vi "SubPanel_DataCollection_Rev11_v12.vi"(0 "DCPowerInformationClusterArray_Input":T7(array[cluster]), 1 "VISAPowerInfoInputArray":T6(array[cluster]), 2 "Run Data SubPanel Input":T5, 3 "RF Block Input Array":T1[](array[typedef]), 4 "Oscilloscope Info Array":T4(array[cluster]) {"vertical coupling" items=["AC", "DC", "Ground"]}, 6 "New Run?":bool, 7 "error in":errorcluster) -> (20 "DCPowerInformationClusterArray_Output":T7(array[cluster]), 21 "VISAPowerInfoInputOutput":T6(array[cluster]), 22 "Run Data SubPanel Output":T5, 23 "RF Subpanel Output":T1[](array[typedef]), 24 "Oscilloscope Info Array Output":T4(array[cluster]) {"vertical coupling" items=["AC", "DC", "Ground"]}, 25 "Reinitialize?":bool, 26 "Data Was Collected?":bool, 27 "error out":errorcluster)   [LabVIEW 2019]
uses:
  Controls/DataBlockControl.ctl
  Controls/QueueDataControl_V3.ctl
  <vilib>/Utility/file.llb/Write Delimited Spreadsheet (string).vi
  Controls/RFBlockControl.ctl
  <instrlib>/niScope/Controls/niScope vertical coupling.ctl
panel:
  out "RFSourceInfoArray":string[][](array[string])
  out "OscilloscopeInfoArray":string[][](array[string])
  out "Voltage Waveform Array":waveform(dbl)[](array[waveform])
  out "Current Waveform Array":waveform(dbl)[](array[waveform])
  out "Current Measurements Live":T2(graph)
  out "Voltage Measurements Live":T2(graph)
  out "DCPowerInfoArray":string[][](array[string])
  out "Current Measurements Total":cluster{dbl[], dbl[]}[](graph)
  out "Voltage Measurements Total":cluster{dbl[], dbl[]}[](graph)
  out "Exiting":bool
  out "Full Run Information":string
  out "Ready For Next Run?":bool
  in  "Next Run":bool
  out "Recording Data":bool
  in  "Record Data Toggle":bool
  out "error of collection":errorcluster
  in  "force exit SubVI":bool
  out "RF Block Parameters Output":T1
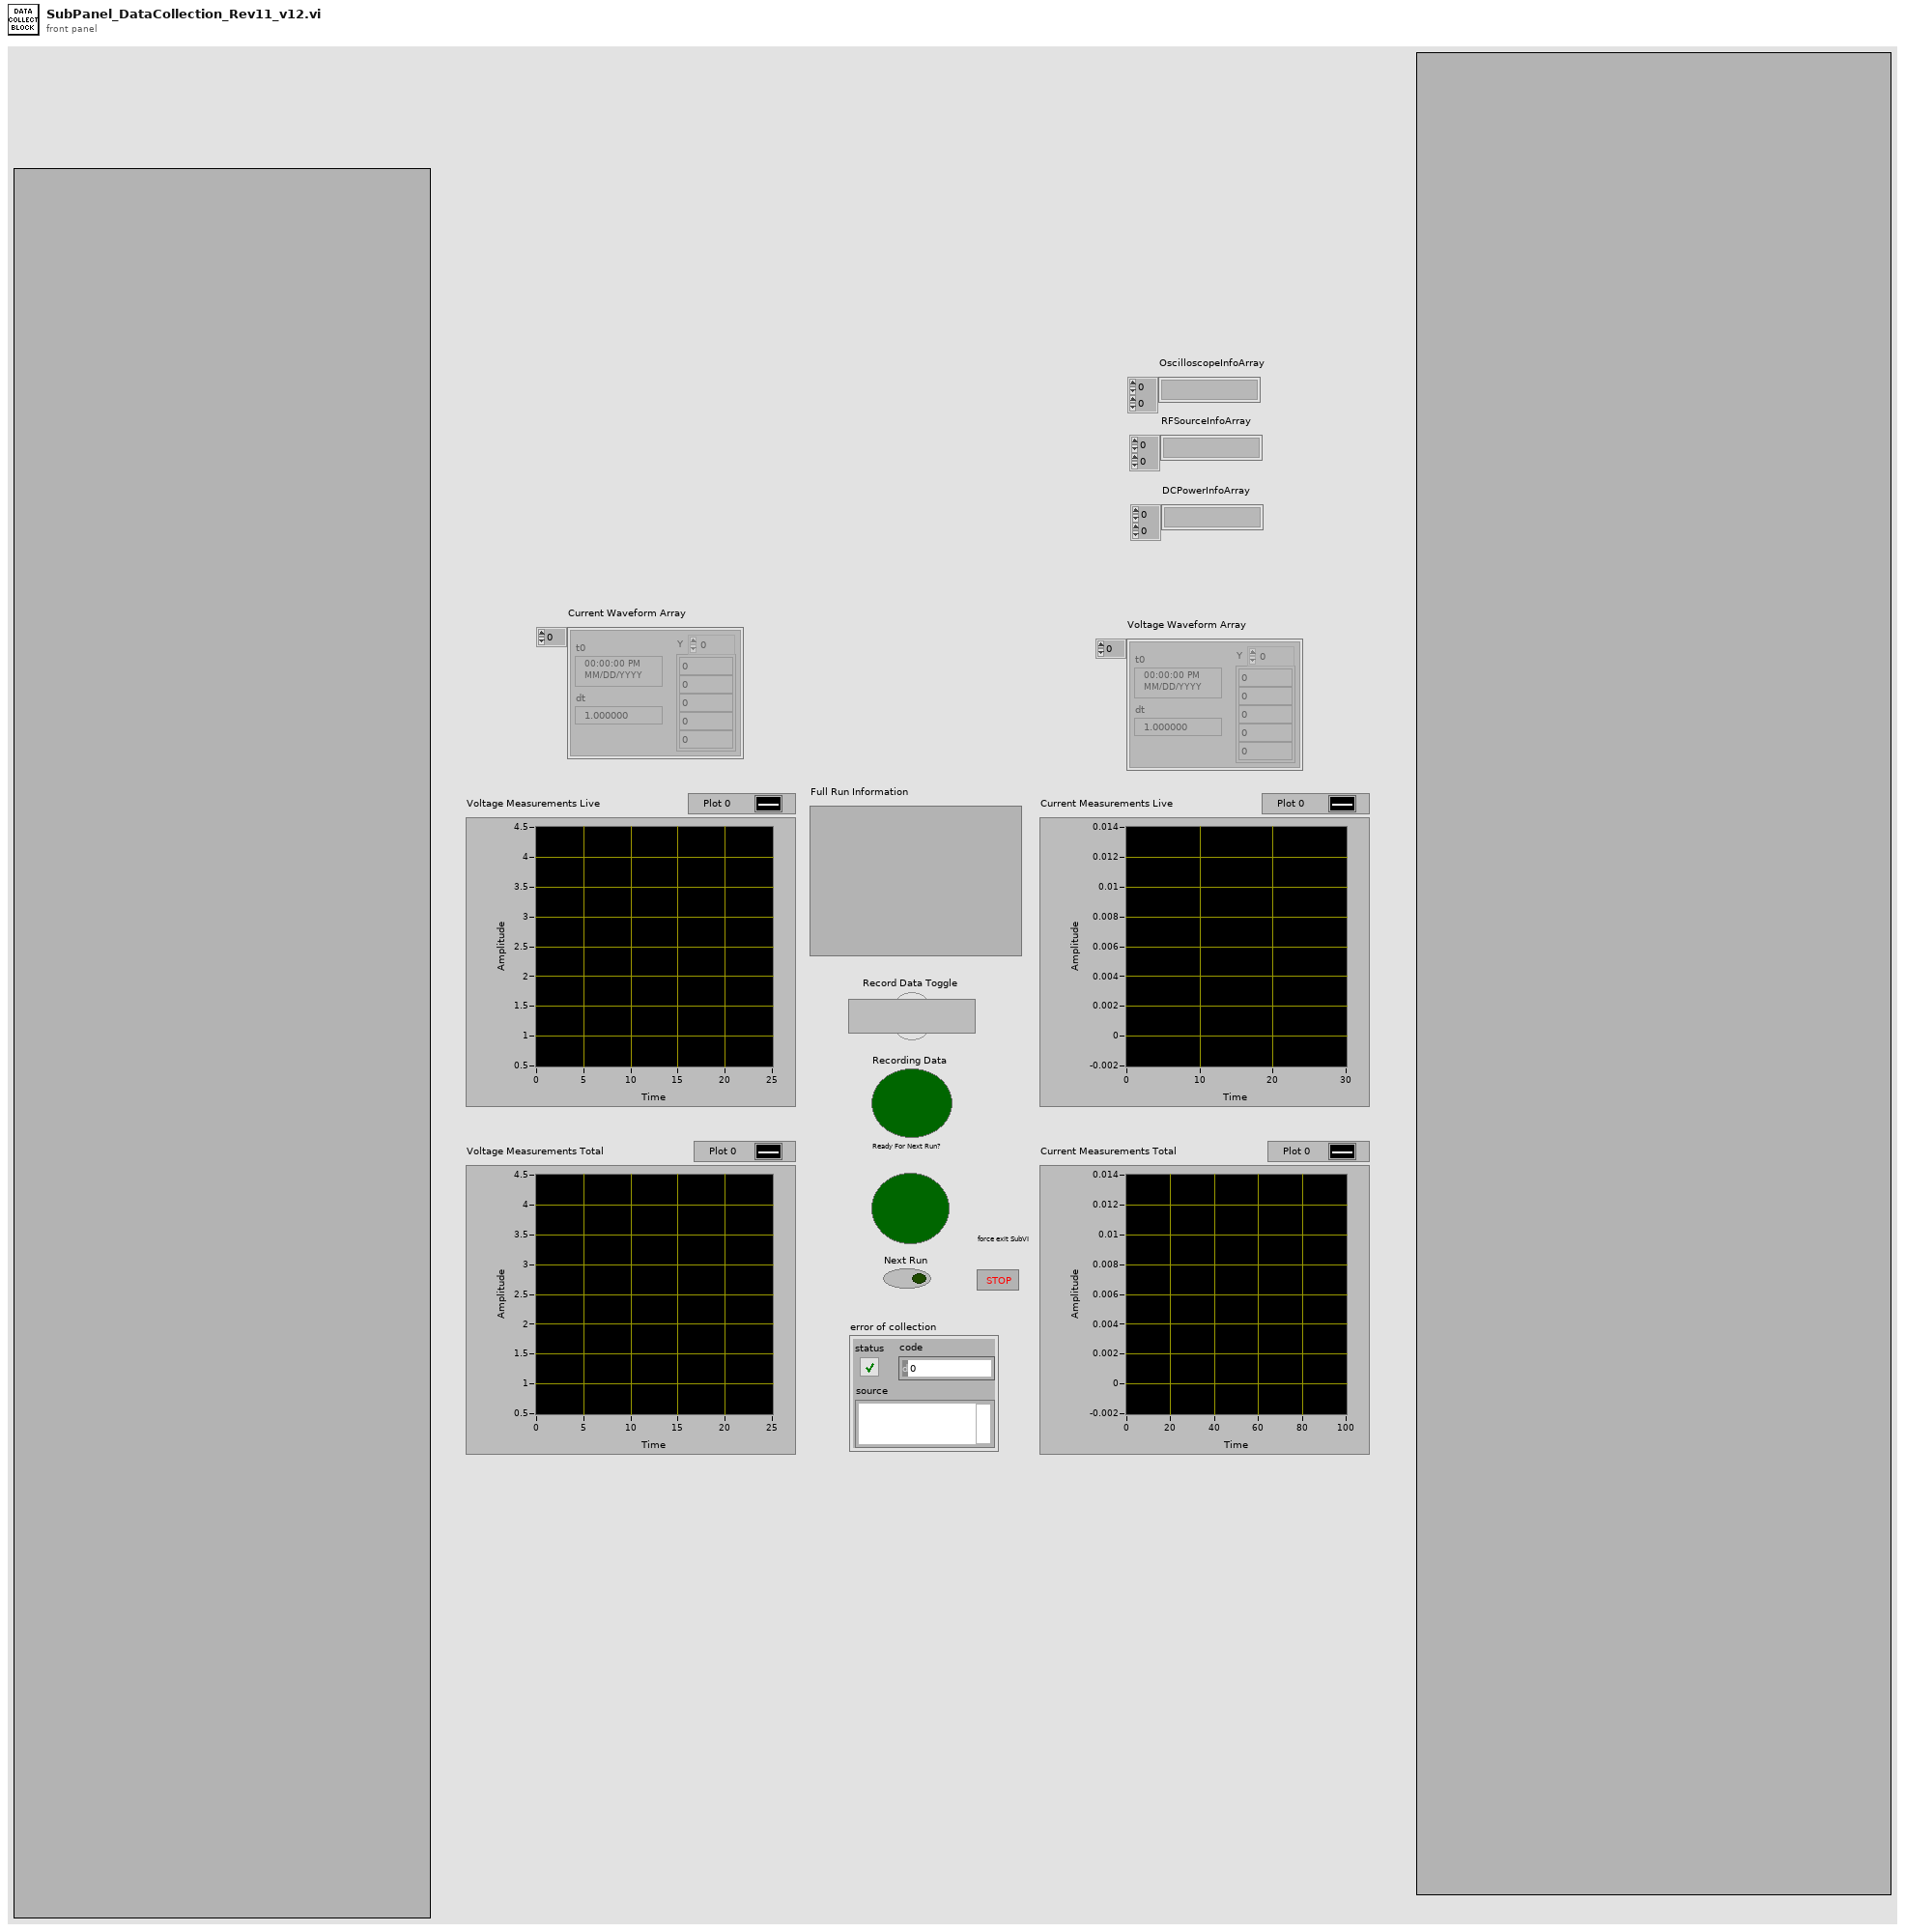
[diagram p1: front panel]
types:
  T1 = typedef "RFBlockControl.ctl" = cluster{"VISA resource name":refnum<visa-resource-name>, "RF Power State In":bool, "Frequency (GHz) Output":dbl, "Power (dBm) Output":dbl, "Instrument Name":string}
  T2 = cluster{"Array of fetched data":dbl[], "Array of fetched data":dbl[]}[]
  T3 = typedef "niScope vertical coupling.ctl" = i32
  T4 = cluster{"instrument handle out":refnum<k15>, "channel numbers array":string[], "channel names array":string[], "vertical range":dbl, "vertical coupling":T3, "Channel 0 50 ohms?":bool, "50 ohm vertical range (V)":dbl, "min record length":i32, "Actual Sample Rate":dbl}[]
  T5 = typedef "DataBlockControl.ctl" = cluster{"Run Folder Parent Directory":path, "DUT":string, "Ion (ex Kr)":string, "Board Number":string, "Effective LET":string, "Test Type":enum16{"Single Event Latchup", "Single Event Transient", "Single Event Upset"}}
  T6 = cluster{"VISA resource name":refnum<visa-resource-name>, "String List":string, string[], "Input Array (Voltage,Current_Limit)":dbl[], "Input Array (Voltage,Current_Limit)":dbl[], "Channel Names":string[], "read buffer":string}[]
  T7 = cluster{"instrument handle out":refnum<k15>, string, string[], dbl[], string[], "Current Limit Output Array":dbl[], dbl[]}[]
  T8 = enum16{"open", "replace", "create", "open or create", "replace or create", "replace or create with confirmation"}
  T9 = typedef "QueueDataControl_V3.ctl" = cluster{"Array of fetched data":dbl[][][], "Channel Names Array":string[], "Voltage Waveform Array":waveform(dbl)[], "Current Waveform Array":waveform(dbl)[], "Resetting Time":timestamp}
  T10 = cluster{"IVI Refnum out":refnum<k15>, string, "voltage level channel 23":dbl, "Channel Name 23":string, "Current Limit":dbl, "Measure Record dt":dbl, string}[]
  T11 = cluster{"created path":path, "DCPowerInformation_byChannel":cluster{"IVI Refnum out":refnum<k15>, string, "voltage level channel 23":dbl, "Channel Name 23":string, "Current Limit":dbl, "Measure Record dt":dbl, string}[], string[]}
  T12 = cluster{"Array of fetched data":dbl[][], string, i32[]}
  T13 = enum16{"Single Event Latchup", "Single Event Transient", "Single Event Upset"}
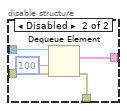
[diagram p3: hidden frame]
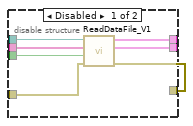
[diagram p5: hidden frame]
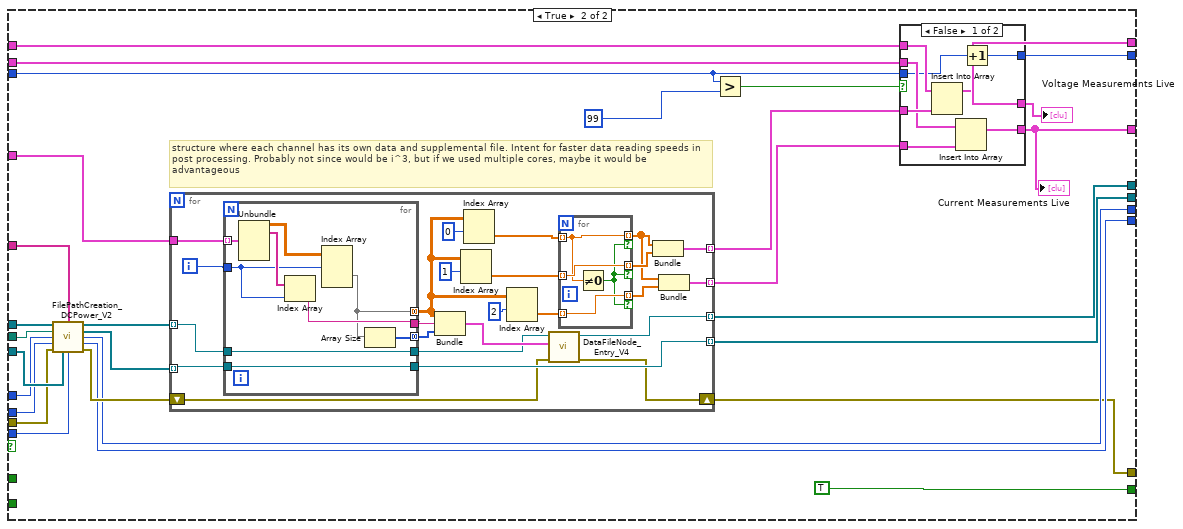
[diagram p6: hidden frame]
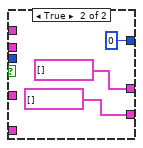
[diagram p7: hidden frame]
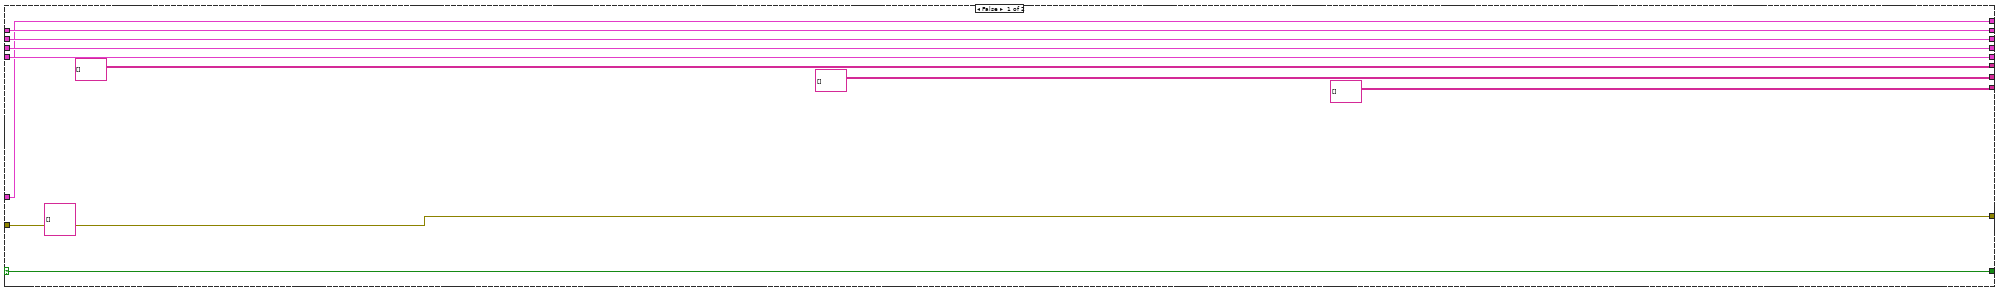
[diagram p8: hidden frame]
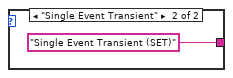
[diagram p9: hidden frame]
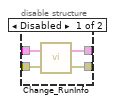
[diagram p13: hidden frame]
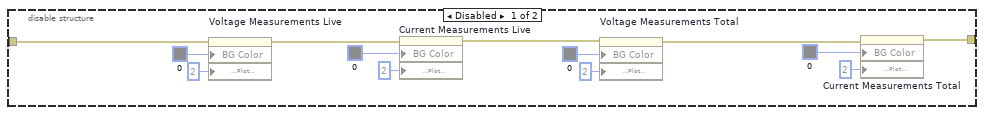
[diagram p14: hidden frame]
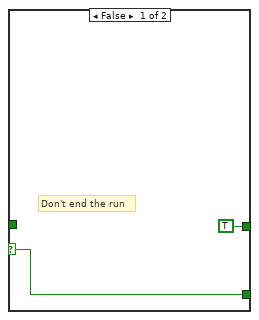
[diagram p16: hidden frame]
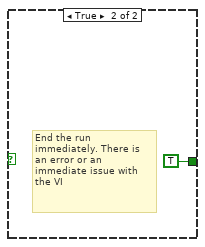
[diagram p17: hidden frame]
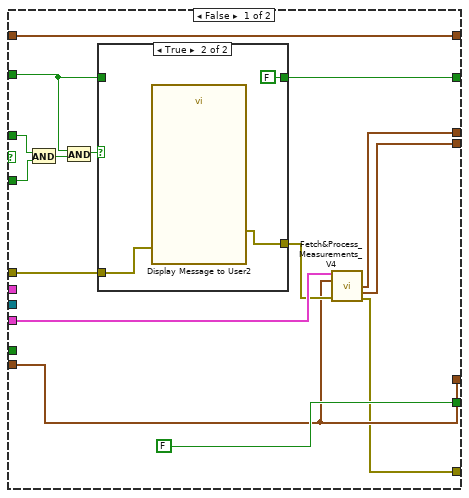
[diagram p19: hidden frame]
diagram:
  (unwired) string[] ["Instrument Name", "Channel Name", "Instrument Channel Number", "Voltage (V)", "Current Limit (A)", "Measure Record delta Time (s)"] ("new element/subarray")
  w76 = T9 {"Array of fetched data"=[], "Channel Names Array"=[], "Voltage Waveform Array"=[], "Current Waveform Array"=[], "Resetting Time"=timestamp(0 s since 1904-01-01)} ("DCPower Queue Data Double Array Format")
  (unwired) T9 {"Array of fetched data"=[], "Channel Names Array"=[], "Voltage Waveform Array"=[], "Current Waveform Array"=[], "Resetting Time"=timestamp(0 s since 1904-01-01)} ("DCPower Double Array Queue")
  (unwired) 10000 ("binary file indexor in")
  (unwired) T5 {"Run Folder Parent Directory"=path "", "DUT"="", "Ion (ex Kr)"="", "Board Number"="", "Effective LET"="", "Test Type"=enum."Single Event Latchup"} ("Run Data Configuration")
  # "Initiating the queue"
  # "echoing run information"
  # "Checking if this is a new run. If it is, a new folder is created along with references to a datafile node. If it is not new (i.e. you didn't start recording data because you needed to make a last minute change and pressed forced exit subvi), the previous folder that is theoretically empty (or just has the .txt files is used"
  # "If yes, you go into this subVI"
  # "This is the message at the beginning confirming if you want to make small changes to the program (i.e. LET)"
  # "Parameters from the configuration stage of this program"
  # "Reset the graph that is saving every 10 seconds of data. Every reset the low bound of the ten seconds is"
  # "Need to change to reflect number of channels that are being recorded. Collect this from a parameters file eventually that will be created"
  # "Indicator if the system is ready for another run. Also indicates if data was actually collected"
  # "Resets the system to start recording"
  # "A flag to ensure the warning message shows only once and doesn't lock the system"
  # "Initiating all of the DC Power instruments (doing this here so because we force abort channels in the DCPower setup because buffer overflow issues. Iterating over the instrument array and the active channel list"
  n1 = flat-sequence {
    tunnel: [w117] -> w92
    tunnel: "error in" -> [w107]
    tunnel: [w121] -> w97
    tunnel: "Run Data SubPanel Input" -> [w109]
    frame #0 {
      n2 = disable-structure shown="Enabled" {
        disable-tunnel: w107 -> [w134 w135]
        disable-tunnel: [w130 w135] -> w106
        frame Disabled {
          n3 = property on="Voltage Measurements Live" class="XYGraph (strict)"(error in=w134, "BG Color"=u32 0 ("Plot.Plot Color"), "Plot.Plot Interpolation"=u8 2) -> (error out=w133:errorcluster)  [unwired: 1 in, 1 out]
          n4 = property on="Current Measurements Live" class="XYGraph (strict)"(error in=w133, "BG Color"=u32 0 ("Plot.Plot Color"), "Plot.Plot Interpolation"=u8 2) -> (error out=w132:errorcluster)  [unwired: 1 in, 1 out]
          n5 = property on="Voltage Measurements Total" class="XYGraph (strict)"(error in=w132, "BG Color"=u32 0 ("Plot.Plot Color"), "Plot.Plot Interpolation"=u8 2) -> (error out=w131:errorcluster)  [unwired: 1 in, 1 out]
          n6 = property on="Current Measurements Total" class="XYGraph (strict)"(error in=w131, "BG Color"=u32 0 ("Plot.Plot Color"), "Plot.Plot Interpolation"=u8 2) -> (error out=w130:errorcluster)  [unwired: 1 in, 1 out]
        }
        frame Enabled {
        }
      }
      n7 = local write "Voltage Measurements Total"(cluster{dbl[], dbl[]}[] [] ("Voltage Measurements")) -> ()
      n8 = local write "Current Measurements Total"(cluster{dbl[], dbl[]}[] [] ("Current Measurements")) -> ()
      n9 = local write "Recording Data"(FALSE ("Recording Data")) -> ()
      n10 = local write "Exiting"(FALSE ("Forced Exit")) -> ()
      n11 = call "Convert_RunInfoCluster_2_RunInfoStringList.vi"("error in"=w106, "Run Number"="", "Run Data SubPanel Input"=w109) -> ("error output"=w110:errorcluster, "Run Data Output"=w111:string)
      n12 = call "Display Message to User"("error in (no error)"=w110, "Enable"=TRUE, "Message"=w111) -> ("error out"=w117:errorcluster)  [unwired: 7 in, 1 out]
      n13 = Two Button Dialog(message="Changing the LET?", 1:"No" ("F button name (\"Cancel\")"), 2:"Yes" ("T button name (\"OK\")")) -> (T button?=w121:bool)
    }
  }
  n14 = call "Convert_InstrumentReferenceArray_2_ChannelReferenceArray.vi"("error in (no error)"=w92, "DCPowerInformationClusterArray_Input"="DCPowerInformationClusterArray_Input") -> ("error out"=w91:errorcluster, "DCPowerInformation_byChannel"=w51:T10)
  n15 = case shown="True" w97 {
    tunnel: "Run Data SubPanel Input" -> [w137 w141]
    tunnel: [w137 w140] -> w29
    tunnel: [w136 w139] -> w93
    tunnel: w91 -> [w136 w138]
    frame False {
    }
    frame True {
      n16 = disable-structure shown="Enabled" {
        disable-tunnel: w141 -> [w145 w147]
        disable-tunnel: [w144 w146] -> w140
        disable-tunnel: [w143 w149] -> w139
        disable-tunnel: w138 -> [w142 w148]
        frame Disabled {
          n17 = call "Change_RunInfo.vi"("error in (no error)"=w142, "Run Data SubPanel in"=w145) -> ("error out"=w143:errorcluster, "Run Data SubPanel out"=w144:T5)
        }
        frame Enabled {
          n18 = call "Change_RunInfo_V2.vi"("error in (no error)"=w148, "Run Data SubPanel in"=w147) -> ("error out"=w149:errorcluster, "Run Data SubPanel out"=w146:T5)
        }
      }
    }
  }
  n19 = Unbundle(w29) -> ("Run Folder Parent Directory"=w94:path)  [unwired: 5 out]
  n20 = List Folder(path=w94, error in=w93) -> (folder names=w95:string[], error out=w79:errorcluster)  [unwired: 2 in, 2 out]
  n21 = Array Size(array=w95) -> (size(s)=w82:i32)
  n22 = case shown="True" "New Run?" {
    selector: "New Run?" -> [w151 w154]
    tunnel: [w152 w156] -> w83
    tunnel: w82 -> [w152 w155]
    tunnel: [w151 w154] -> w81
    tunnel: [w150 w153] -> w80
    tunnel: w79 -> [w150 w153]
    frame False {
    }
    frame True {
      n23 = Increment(x=w155) -> (x+1=w156:i32)
    }
  }
  n24 = Number To Decimal String(number=w83) -> (decimal integer string=w86:string)  [unwired: 1 in]
  n25 = Concatenate Strings("Run_", w86) -> (w28:string)
  n26 = Array Size(array=w51) -> (size(s)=w78:i32)
  n27 = call "InitialFileFolderCreation_V2.vi"("New Run?"=w81, "error in (no error)"=w80, "Run Number"=w28, "DCPowerArrayClusterSize"=w78, "base path"=w94) -> ("error out"=w27:errorcluster, "SupplementalDataFileReferenceObjectArray"=w89:refnum<file>[], "DataFileReferenceObjectArray"=w90:refnum<file>[], "created path"=w36:path)  [unwired: 3 in]
  n28 = call "Convert_RunInfoCluster_2_RunInfoStringList.vi"("error in"=w27, "Run Number"=w28, "Run Data SubPanel Input"=w29) -> ("error output"=w26:errorcluster, "Run Data Output"=→"Full Run Information":string)
  n29 = for {
    shift-right: [w157] -> w34
    shift-left: w26 -> [w159]
    tunnel: "DCPowerInformationClusterArray_Input" -> [w161] mode=indexing
    n30 = Unbundle(w161) -> ("instrument handle out"=w158:refnum<k15>, w160:string)  [unwired: 5 out]
    n31 = call <instrlib>:"niDCPower Initiate With Channels.vi"("error in (no error)"=w159, "channel name"=w160, "instrument handle"=w158) -> ("error out"=w157:errorcluster)  [unwired: 7 in, 1 out]
  }
  n32 = disable-structure shown="Enabled" {
    disable-tunnel: w34 -> [w165 w167]
    disable-tunnel: [w164 w167] -> w31
    disable-tunnel: [w163 _] -> w102
    disable-tunnel: w76 -> [w162 _]
    frame Enabled {
      n33 = Obtain Queue(name (unnamed)="DCPowerQueue", element data type=w162, error in (no error)=w165) -> (queue out=w163:refnum<queue>, error out=w164:errorcluster)  [unwired: 2 in, 1 out]
    }
    frame Disabled {
    }
  }
  n34 = disable-structure shown="Disabled" {
    frame Disabled {
      n35 = Reshape Array() -> ()  [unwired: 2 in, 1 out]
    }
    frame Enabled {
    }
  }
  n36 = for {
    tunnel: w51 -> [w169] mode=indexing
    tunnel: [w168] -> w52 mode=indexing
    # "Creating Array of Channel Names"
    n37 = Unbundle(w169) -> ("Channel Name 23"=w168:string)  [unwired: 6 out]
  }
  n38 = Bundle("created path"=w36, "DCPowerInformation_byChannel"=w51, w52) -> (w50:T11)  [unwired: 1 in]
  n39 = Array Size(array=w52) -> (size(s)=w71:i32)
  n40 = Get Date/Time In Seconds() -> (seconds since 1Jan1904=w32:timestamp)
  n41 = while {
    tunnel: w102 -> [w202]
    shift-right: [w189] -> w73
    shift-left: w31 -> [w201]
    tunnel: w36 -> [w198]
    shift-right: [w191] -> w75
    shift-left: w90 -> [w199]
    shift-right: [w190] -> w74
    shift-left: w89 -> [w197]
    shift-right: [w193] -> _
    shift-left: 0 ("binary file indexor in") -> [w196]
    shift-right: [w192] -> _
    shift-left: 0 ("binary file indexor in") -> [w195]
    tunnel: 1000 ("binary file indexor in") -> [w194]
    tunnel: w52 -> [w200]
    tunnel: w71 -> [_]
    shift-right: [w178] -> _
    shift-left: FALSE -> [w177]
    shift-right: [w174] -> _
    shift-left: T2 [] ("array") -> [w175]
    shift-right: [w172] -> _
    shift-left: T2 [] ("array") -> [w173]
    shift-right: [w170] -> _
    shift-left: 0 -> [w171]
    stop <- w186 stop-if-true
    # "If recording data is on, there should always be elements in the queue, so I shouldn't have to worry about a state where the \"recording data\" is active but there is no data in the queue, if so, then I'll just have to find an alternative to the OR statement"
    n42 = Get Queue Status(queue=w202, error in (no error)=w201) -> (queue out=w183:refnum<queue>, error out=w184:errorcluster, # elements in queue=w179:i32)  [unwired: 1 in, 5 out]
    n43 = local read "Recording Data"() -> (w176:bool)
    n44 = disable-structure shown="Enabled" {
      disable-tunnel: [w206 w208] -> w185
      disable-tunnel: w184 -> [w205 w210]
      disable-tunnel: w183 -> [w204 w211]
      disable-tunnel: [w203 w207] -> w182
      frame Enabled {
        n45 = Flush Queue(queue=w204, error in (no error)=w205) -> (remaining elements=w203:T9[], error out=w206:errorcluster)  [unwired: 1 out]
      }
      frame Disabled {
        n46 = Dequeue Element(queue=w211, timeout in ms (-1)=100, error in (no error)=w210) -> (element=w207:T9, error out=w208:errorcluster)  [unwired: 2 out]
      }
    }
    n47 = Not Equal To 0?(x=w179) -> (x != 0?=w181:bool)
    n48 = And(x=w181, y=w176) -> (x .and. y?=w180:bool)
    n49 = case shown="False" w180 {
      tunnel: w182 -> [_ w289]
      tunnel: w185 -> [w219 w283]
      tunnel: w200 -> [w220 w275]
      tunnel: w199 -> [w227 w288]
      tunnel: w198 -> [w221 w287]
      tunnel: w197 -> [w228 w286]
      tunnel: w196 -> [w226 w285]
      tunnel: w195 -> [w225 w274]
      tunnel: w194 -> [_ w273]
      tunnel: [w226 w282] -> w193
      tunnel: [w225 w281] -> w192
      tunnel: [w227 w278] -> w191
      tunnel: [w228 w277] -> w190
      tunnel: [w218 w276] -> w189
      tunnel: [w217 TRUE] -> w178
      tunnel: w177 -> [w216 _]
      tunnel: w176 -> [w224 _]
      tunnel: w175 -> [w215 w269]
      tunnel: [w215 w268] -> w174
      tunnel: w173 -> [w214 w267]
      tunnel: [w214 w266] -> w172
      tunnel: w171 -> [w213 w263]
      tunnel: [w212 w262] -> w170
      frame False {
        n50 = Not(x=w224) -> (.not. x?=w223:bool)
        n51 = And(x=w223, y=w216) -> (x .and. y?=w222:bool)
        n52 = case shown="True" w222 {
          tunnel: w221 -> [_ w240]
          tunnel: w220 -> [_ w239]
          tunnel: w219 -> [w231 w237]
          tunnel: [w231 w236] -> w218
          tunnel: [w230 FALSE] -> w217
          tunnel: w216 -> [w230 _]
          tunnel: w213 -> [w229 _]
          tunnel: [w229 0] -> w212
          frame False {
          }
          frame True {
            n53 = disable-structure shown="Enabled" {
              disable-tunnel: w240 -> [w247 w252]
              disable-tunnel: w239 -> [w246 w251]
              disable-tunnel: FALSE ("Create CSV files?") -> [w245 w253]
              disable-tunnel: w237 -> [w244 w254]
              disable-tunnel: [w243 _] -> w236
              disable-tunnel: [w242 w249] -> w234
              disable-tunnel: [w241 w248] -> w233
              frame Disabled {
                n54 = call "ReadDataFile_V1.vi"("error in (no error)"=w244, "Create CSV files?"=w245, "Channel Names Array"=w246, "DataFolder Path"=w247) -> ("error out"=w243:errorcluster, "Current Measurements"=w241:cluster{dbl[], dbl[]}[], "Voltage Measurements"=w242:cluster{dbl[], dbl[]}[])  [unwired: 5 in]
              }
              frame Enabled {
                n55 = Array Size(array=w251) -> (size(s)=w250:i32)
                n56 = for {
                  tunnel: w254 -> [w261]
                  tunnel: w253 -> [w260]
                  tunnel: w252 -> [w259]
                  tunnel: w251 -> [w258] mode=indexing
                  tunnel: w250 -> [w257]
                  tunnel: [w256] -> w249 mode=indexing
                  tunnel: [w255] -> w248 mode=indexing
                  n57 = call "ReadDataFile_V2.vi"("Channel Name Array Size"=w257, "error in (no error)"=w261, "Create CSV files?"=w260, "Channel Name Individual"=w258, "DataFolder Path"=w259) -> ("Current Measurements Individual"=w255:cluster{dbl[], dbl[]}, "Voltage Measurements Individual"=w256:cluster{dbl[], dbl[]})  [unwired: 4 in, 1 out]
                }
              }
            }
            "Voltage Measurements Total" <- w234
            "Current Measurements Total" <- w233
          }
        }
      }
      frame True {
        # "structure where each channel has its own data and supplemental file. Intent for faster data reading speeds in post processing. Probably not since would be i^3, but if we used multiple cores, maybe it would be advantageous"
        n58 = call "FilePathCreation_DCPower_V2.vi"("binary file input reference array 1"=w288, "Channel Name Input array"=w275, "data output directory folder"=w287, "binary file indexor in"=w285, "Reset counter in"=w274, "error in (no error)"=w283, "binary file input reference array 2"=w286, "reset threshold"=w273) -> ("binary file output reference array"=w280:refnum<file>[], "binary file output reference array 2"=w279:refnum<file>[], "binary file indexor out"=w282:i32, "reset counter out"=w281:i32, "error out"=w284:errorcluster)  [unwired: 3 in]
        n59 = for {
          shift-right: [w314] -> w276
          shift-left: w284 -> [w315]
          tunnel: w289 -> [w324]
          tunnel: w279 -> [w321] mode=indexing
          tunnel: w280 -> [w320] mode=indexing
          tunnel: [w319] -> w277 mode=indexing
          tunnel: [w313] -> w278 mode=indexing
          tunnel: [w308] -> w271 mode=indexing
          tunnel: [w307] -> w270 mode=indexing
          i -> [w318]
          n60 = for {
            tunnel: w324 -> [w337] mode=indexing
            tunnel: w318 -> [w334]
            tunnel: [w329] -> w309 mode=concatenating
            tunnel: [w333] -> w323
            tunnel: w321 -> [w332]
            tunnel: w320 -> [w330]
            tunnel: [w330] -> w316
            tunnel: [w332] -> w319
            tunnel: [w331] -> w322 mode=concatenating
            n61 = Unbundle(w337) -> ("Array of fetched data"=w336:dbl[][][], "Channel Names Array"=w335:string[])  [unwired: 3 out]
            n62 = Index Array(array=w335, index=w334) -> (element=w333:string)
            n63 = Index Array(array=w336, index (dim 0)=w334) -> (element=w329:dbl[][])  [unwired: 2 in]
            n64 = Array Size(array=w329) -> (size(s)=w331:i32[])
          }
          n65 = Bundle("Array of fetched data"=w309, w323, w322) -> (w317:T12)  [unwired: 1 in]
          n66 = Index Array(array=w309, index (row)=1) -> (element=w304:dbl[])  [unwired: 1 in]
          n67 = Index Array(array=w309, index (row)=0) -> (element=w306:dbl[])  [unwired: 1 in]
          n68 = Index Array(array=w309, index (row)=2) -> (element=w302:dbl[])  [unwired: 1 in]
          n69 = call "DataFileNode_Entry_V4.vi"("error in (no error)"=w315, "Queued Elements"=w317, "Byte Stream File in"=w316) -> ("error out"=w314:errorcluster, "Byte Stream File out"=w313:refnum<file>)  [unwired: 7 in]
          n70 = for {
            tunnel: [w326] -> w301 mode=indexing if=w325
            tunnel: w306 -> [w326] mode=indexing
            tunnel: [w328] -> w305 mode=indexing if=w325
            tunnel: w304 -> [w328] mode=indexing
            tunnel: [w327] -> w303 mode=indexing if=w325
            tunnel: w302 -> [w327] mode=indexing
            n71 = Not Equal To 0?(x=w326) -> (x != 0?=w325:bool)
          }
          n72 = Bundle(w301, w305) -> (w308:cluster{dbl[], dbl[]})  [unwired: 1 in]
          n73 = Bundle(w301, w303) -> (w307:cluster{dbl[], dbl[]})  [unwired: 1 in]
        }
        n74 = Greater?(x=w263, y=99) -> (0:w265:bool)
        n75 = case shown="False" w265 {
          tunnel: w271 -> [w297 _]
          tunnel: w270 -> [w296 _]
          tunnel: w269 -> [w295 _]
          tunnel: [w294 T2 [] ("array")] -> w268
          tunnel: w267 -> [w293 _]
          tunnel: [w292 T2 [] ("array")] -> w266
          tunnel: w263 -> [w291 _]
          tunnel: [w290 0] -> w262
          frame False {
            n76 = Insert Into Array(array=w295, new element=w297) -> (w294:T2)  [unwired: 1 in]
            n77 = Insert Into Array(array=w293, new element=w296) -> (w292:T2)  [unwired: 1 in]
            n78 = Increment(x=w291) -> (x+1=w290:i32)
          }
          frame True {
          }
        }
        "Voltage Measurements Live" <- w268
        "Current Measurements Live" <- w266
      }
    }
    n79 = local read "Exiting"() -> (w188:bool)
    n80 = Equal To 0?(x=w179) -> (x = 0?=w187:bool)
    n81 = And(x=w187, y=w188) -> (x .and. y?=w186:bool)
  }
  n82 = while {
    shift-right: [w368] -> w40
    shift-left: "DCPowerInformationClusterArray_Input" -> [w368]
    shift-right: [w372] -> w42
    shift-left: "VISAPowerInfoInputArray" -> [w372]
    shift-right: [w371] -> w44
    shift-left: w29 -> [w371]
    shift-right: [w370] -> w46
    shift-left: "RF Block Input Array" -> [w370]
    shift-right: [w369] -> w48
    shift-left: "Oscilloscope Info Array" -> [w369]
    shift-right: [w355] -> w77
    shift-left: w31 -> [w366]
    tunnel: w51 -> [w367]
    shift-right: [w365] -> _
    shift-left: FALSE -> [w362]
    tunnel: w102 -> [w364]
    shift-right: [w344] -> _
    shift-left: FALSE -> [w349]
    tunnel: [w353] -> w101
    shift-right: [w347] -> _
    shift-left: TRUE ("x .and. y?") -> [w348]
    shift-right: [w345] -> _
    shift-left: w32 -> [w346]
    tunnel: [w344] -> w39
    tunnel: w76 -> [w342]
    shift-right: [w339] -> w19
    shift-left: timestamp(0 s since 1904-01-01) ("seconds since 1Jan1904") -> [w338]
    stop <- w343 stop-if-true
    # "If I am going to reset the entire configuration or if we are going up in LET only. True, reset the system. False, don't reset the system"
    n83 = Not(x=w349) -> (.not. x?=w351:bool)
    n84 = And(x="Record Data Toggle", y=w351) -> (x .and. y?=w352:bool)
    "Recording Data" <- w352
    n85 = case shown="True" w352 {
      tunnel: w367 -> [w401 w416]
      tunnel: w366 -> [w399 w423]
      tunnel: [w389 w411] -> w341
      tunnel: [w390 w410] -> w340
      tunnel: w362 -> [_ w421]
      tunnel: [FALSE w422] -> w365
      tunnel: w364 -> [_ w420]
      tunnel: [w388 w419] -> w360
      tunnel: "Record Data Toggle" -> [w396 _]
      tunnel: w349 -> [w397 _]
      tunnel: w348 -> [w392 _]
      tunnel: [w393 TRUE] -> w347
      tunnel: w346 -> [w391 w424]
      tunnel: [w391 w414] -> w345
      tunnel: w342 -> [_ w418]
      tunnel: [w387 w408] -> w339
      tunnel: w338 -> [w387 w407]
      frame False {
        n86 = And(x=w396, y=w397) -> (x .and. y?=w395:bool)
        n87 = And(x=w392, y=w395) -> (x .and. y?=w394:bool)
        n88 = case shown="True" w394 {
          tunnel: [w403 w405] -> w398
          tunnel: w399 -> [w403 w406]
          tunnel: [w402 FALSE] -> w393
          tunnel: w392 -> [w402 _]
          frame False {
          }
          frame True {
            n89 = call "Display Message to User2"("error in (no error)"=w406) -> ("error out"=w405:errorcluster)  [unwired: 9 in, 1 out]
          }
        }
        n90 = call "Fetch&Process_Measurements_V4.vi"("DCPowerInformation_byChannel"=w401, "Initial Time"=w391, "error in (no error)"=w398) -> ("Current Waveform Array"=w389:waveform(dbl)[], "Voltage Waveform Array"=w390:waveform(dbl)[], "error out"=w388:errorcluster)  [unwired: 6 in, 4 out]
      }
      frame True {
        n91 = case shown="True" w421 {
          tunnel: [w426 w432] -> w414
          tunnel: w424 -> [_ w432]
          tunnel: w423 -> [w427 w431]
          tunnel: [w427 w431] -> w415
          tunnel: [TRUE w430] -> w422
          tunnel: w421 -> [_ w430]
          tunnel: [w426 w429] -> w408
          tunnel: w407 -> [_ w429]
          frame False {
            n92 = Get Date/Time In Seconds() -> (seconds since 1Jan1904=w426:timestamp)
          }
          frame True {
          }
        }
        n93 = call "Fetch&Process_Measurements_V4.vi"("DCPowerInformation_byChannel"=w416, "Initial Time"=w414, "error in (no error)"=w415) -> ("Data As dbl Array"=w413:dbl[][][], "Channel Number Array"=w412:string[], "Current Waveform Array"=w411:waveform(dbl)[], "Voltage Waveform Array"=w410:waveform(dbl)[], "error out"=w409:errorcluster)  [unwired: 6 in, 2 out]
        n94 = Bundle(cluster=w418, "Array of fetched data"=w413, "Channel Names Array"=w412) -> (w417:T9)  [unwired: 3 in]
        n95 = Enqueue Element(queue=w420, element=w417, error in (no error)=w409) -> (error out=w419:errorcluster)  [unwired: 1 in, 2 out]
      }
    }
    "Current Waveform Array" <- w341
    "Voltage Waveform Array" <- w340
    n96 = Not(x=w352) -> (.not. x?=w363:bool)
    n97 = And(x=w363, y=w362) -> (x .and. y?=w361:bool)
    n98 = case shown="True" w361 {
      tunnel: w360 -> [w383 w385]
      tunnel: [w384 TRUE] -> w344
      tunnel: w349 -> [w384 _]
      tunnel: [w383 w385] -> w355
      frame False {
      }
      frame True {
      }
    }
    "error of collection" <- w355
    "Ready For Next Run?" <- w344
    n99 = Or(x=w355, y="force exit SubVI") -> (x .or. y?=w357:bool)
    n100 = And(x="Next Run", y=w344) -> (x .and. y?=w359:bool)
    n101 = Or(x=w357, y=w359) -> (x .or. y?=w358:bool)
    n102 = case shown="True" w358 {
      selector: w358 -> [w374 _]
      tunnel: w357 -> [_ w377]
      tunnel: [w374 TRUE] -> w343
      tunnel: [TRUE ("T button?") w375] -> w353
      frame False {
        # "Don't end the run"
      }
      frame True {
        n103 = case shown="False" w377 {
          tunnel: [w378 TRUE] -> w375
          frame False {
            # "Option to continue the run as is or reset for a new configuration"
            n104 = Two Button Dialog(message="Would you like to change parameters before the next run? ( you will have an option to change LET and board number regardless) ", 1:"No, I may only want to change LET or board number" ("F button name (\"Cancel\")"), 2:"Yes, I want to make changes " ("T button name (\"OK\")")) -> (T button?=w378:bool)
          }
          frame True {
            # "End the run immediately. There is an error or an immediate issue with the VI"
          }
        }
      }
    }
    "Exiting" <- w343
  }
  "Reinitialize?" <- w101
  n105 = for {
    tunnel: w75 -> [w437] mode=indexing
    tunnel: w74 -> [w435] mode=indexing
    shift-right: [w433] -> w72
    shift-left: w73 -> [w436]
    n106 = Close File(refnum=w437, error in=w436) -> (error out=w434:errorcluster)  [unwired: 1 out]
    n107 = Close File(refnum=w435, error in=w434) -> (error out=w433:errorcluster)  [unwired: 1 out]
  }
  n108 = Merge Errors(w77, w72) -> (w54:errorcluster)
  n109 = Unbundle(w50) -> ("created path"=w35:path)  [unwired: 2 out]
  n110 = case shown="True" w39 {
    selector: w39 -> [w442 w547]
    tunnel: w54 -> [w441 w553]
    tunnel: [w441 w452] -> w53
    tunnel: [w447 w484] -> w49
    tunnel: w48 -> [w447 w552]
    tunnel: [w446 w486] -> w47
    tunnel: w46 -> [w446 w551]
    tunnel: [w445 w472] -> w45
    tunnel: w44 -> [w445 w550]
    tunnel: [w444 w489] -> w43
    tunnel: w42 -> [w444 w549]
    tunnel: [w443 w491] -> w41
    tunnel: w40 -> [w443 w548]
    tunnel: [w442 w547] -> w38
    tunnel: [string[][] [] ("DCPowerInfoArray") w482] -> w37
    tunnel: w35 -> [_ w450]
    tunnel: [string[][] [] ("DCPowerInfoArray") w480] -> w3
    tunnel: [string[][] [] ("DCPowerInfoArray") w474] -> w2
    frame False {
      (unwired) string[][][] []
    }
    frame True {
      # "This will be indexed eventually"
      n111 = for {
        shift-right: [w633] -> w543
        shift-left: w553 -> [w645]
        tunnel: w548 -> [w636] mode=indexing
        shift-right: [w644] -> w522
        shift-left: w552 -> [w644]
        shift-right: [w643] -> w521
        shift-left: w551 -> [w643]
        shift-right: [w642] -> w520
        shift-left: w550 -> [w642]
        shift-right: [w641] -> w519
        shift-left: w549 -> [w641]
        shift-right: [w640] -> w518
        shift-left: w548 -> [w640]
        shift-right: [w638] -> w523
        shift-left: string[][] [] ("DCPowerInfoArray") -> [w639]
        # "This puts all the instruments together in one output"
        n112 = Unbundle(w636) -> ("instrument handle out"=w647:refnum<k15>, w646:string)  [unwired: 5 out]
        n113 = call <instrlib>:"niDCPower Abort With Channels.vi"("error in (no error)"=w645, "channel name"=w646, "instrument handle"=w647) -> ("error out"=w634:errorcluster)  [unwired: 7 in, 1 out]
        n114 = call "DCPower_ParameterCreation.vi"("error in"=w634, "Precision"="8", "DCPowerInformationByInstrument"=w636) -> ("error out"=w633:errorcluster, "DCPowerInfoArray"=w632:string[][])
        n115 = Insert Into Array(array=w639, index (col)=0 ("disabled index (col)"), new element=w632) -> (w638:string[][])  [unwired: 1 in]
      }
      n116 = Concatenate Strings("Channel Name " ("string")) -> (w535:string)
      n117 = Concatenate Strings("Voltage (V) " ("string")) -> (w537:string)
      n118 = Concatenate Strings("Measure Record delta Time (s) " ("string")) -> (w539:string)
      n119 = Concatenate Strings("Instrument Name " ("string")) -> (w534:string)
      n120 = Concatenate Strings("Instrument Channel Number " ("string")) -> (w536:string)
      n121 = Concatenate Strings("Current Limit (A) " ("string")) -> (w538:string)
      n122 = Build Array(w534, w535, w536, w537, w538, w539) -> (w527:string[])
      n123 = Build Path(base path=w450, name or relative path="DCPOW_Params.csv") -> (appended path=w542:path)
      n124 = Insert Into Array(array=w523, index (col)=0 ("disabled index (col)"), new element=w527) -> (w526:string[][])  [unwired: 1 in]
      n125 = call-poly <vilib>:"Write Delimited Spreadsheet.vi"("file path (dialog if empty)"=w542, "format (%s)"="%s" ("format (%.3f)"), "2D data"=w526, "error in (no error)"=w543, "transpose? (no:F)"=TRUE, "delimiter (\\t)"="," ("delimiter (\\t)")) -> ("error out"=w524:errorcluster)  [unwired: 8 in, 1 out]
      n126 = for {
        shift-right: [w626] -> w504
        shift-left: w524 -> [w626]
        shift-right: [w621] -> w492
        shift-left: w518 -> [w621]
        shift-right: [w622] -> w490
        shift-left: w519 -> [w622]
        shift-right: [w623] -> w488
        shift-left: w520 -> [w623]
        shift-right: [w624] -> w487
        shift-left: w521 -> [w624]
        shift-right: [w625] -> w483
        shift-left: w523 -> [w625]
        tunnel: w522 -> [w620] mode=indexing
        tunnel: [w620] -> w485 mode=indexing
        shift-right: [w589] -> w481
        shift-left: string[][] [] ("DCPowerInfoArray") -> [w595]
        n127 = Unbundle(w620) -> ("instrument handle out"=w619:refnum<k15>, "channel numbers array"=w592:string[], "channel names array"=w593:string[], "vertical range"=w614:dbl, "vertical coupling"=w608:T3, "Channel 0 50 ohms?"=w613:bool, "50 ohm vertical range (V)"=w612:dbl, "min record length"=w607:i32, "Actual Sample Rate"=w606:dbl)
        n128 = Array Size(array=w592) -> (size(s)=w615:i32)
        n129 = Initialize Array(w614, w615) -> (w611:dbl[])
        n130 = Decimal String To Number(string="8") -> (number=w590:i32)  [unwired: 2 in, 1 out]
        n131 = case shown="True" w613 {
          tunnel: w612 -> [_ w629]
          tunnel: w611 -> [w627 w631]
          tunnel: [w627 w628] -> w610
          frame False {
          }
          frame True {
            n132 = Replace Array Subset(array=w631, new element=w629, index=0) -> (w628:dbl[])
          }
        }
        n133 = Number To Fractional String(number=w606, precision (6)=w590) -> (F-format string=w600:string)  [unwired: 2 in]
        n134 = Number To Decimal String(number=w607) -> (decimal integer string=w601:string)  [unwired: 1 in]
        n135 = Concatenate Strings(w619) -> (w617:string)
        n136 = Number To Fractional String(number=w610, precision (6)=w590) -> (F-format string=w609:string[])  [unwired: 2 in]
        n137 = Number To Decimal String(number=w608) -> (decimal integer string=w602:string)  [unwired: 1 in]
        n138 = Array Size(array=w592) -> (size(s)=w618:i32)
        n139 = Initialize Array(w617, w618) -> (w616:string[])
        n140 = Array Size(array=w592) -> (size(s)=w605:i32)
        n141 = Array Size(array=w592) -> (size(s)=w603:i32)
        n142 = Array Size(array=w592) -> (size(s)=w604:i32)
        n143 = Initialize Array(w602, w605) -> (w599:string[])
        n144 = Initialize Array(w600, w603) -> (w597:string[])
        n145 = Initialize Array(w601, w604) -> (w598:string[])
        n146 = Build Array(w616, w593, w592, w609, w599, w598, w597) -> (w594:string[][])
        n147 = Insert Into Array(array=w595, index (col)=0 ("disabled index (col)"), new element=w594) -> (w589:string[][])  [unwired: 1 in]
      }
      n148 = Build Array("Instrument Name " ("string"), "Channel Name" ("element"), "Instrument Channel Number" ("element"), "Vertical Range (V)" ("element"), "Vertical Coupling" ("element"), "Min Record Length" ("element"), "Actual Sample Rate" ("element")) -> (w508:string[])
      n149 = Insert Into Array(array=w481, index (col)=0 ("disabled index (col)"), new element=w508) -> (w501:string[][])  [unwired: 1 in]
      n150 = Build Path(base path=w450, name or relative path="Oscilloscope_Params.csv") -> (appended path=w506:path)
      n151 = call-poly <vilib>:"Write Delimited Spreadsheet.vi"("file path (dialog if empty)"=w506, "format (%s)"="%s" ("format (%.3f)"), "2D data"=w501, "error in (no error)"=w504, "transpose? (no:F)"=TRUE, "delimiter (\\t)"="," ("delimiter (\\t)")) -> ("error out"=w499:errorcluster)  [unwired: 8 in, 1 out]
      n152 = for {
        shift-right: [w571] -> w497
        shift-left: string[][] [] ("DCPowerInfoArray") -> [w572]
        tunnel: w487 -> [w587] mode=indexing
        shift-right: [w556] -> w473
        shift-left: w499 -> [w563]
        shift-right: [w564] -> w480
        shift-left: w481 -> [w564]
        shift-right: [w565] -> w482
        shift-left: w483 -> [w565]
        shift-right: [w566] -> w484
        shift-left: w485 -> [w566]
        shift-right: [w567] -> w486
        shift-left: w487 -> [w567]
        shift-right: [w568] -> w472
        shift-left: w488 -> [w568]
        shift-right: [w569] -> w489
        shift-left: w490 -> [w569]
        shift-right: [w570] -> w491
        shift-left: w492 -> [w570]
        n153 = Unbundle(w587) -> ("VISA resource name"=w586:refnum<visa-resource-name>, "Frequency (GHz) Output"=w580:dbl, "Power (dBm) Output"=w577:dbl)  [unwired: 2 out]
        n154 = Decimal String To Number(string="8") -> (number=w575:i32)  [unwired: 2 in, 1 out]
        n155 = VISA Write(VISA resource name=w586, write buffer="*IDN?", error in (no error)=w563) -> (VISA resource name out=w582:refnum<visa-resource-name>, return count=w584:u32, error out=w588:errorcluster)
        n156 = Number To Fractional String(number=w577, precision (6)=w575) -> (F-format string=w578:string)  [unwired: 2 in]
        n157 = Add(x=w584, y=u32 10) -> (x+y=w581:u32)
        n158 = Number To Fractional String(number=w580, precision (6)=w575) -> (F-format string=w579:string)  [unwired: 2 in]
        n159 = VISA Read(VISA resource name=w582, byte count=w581, error in (no error)=w588) -> (read buffer=w562:string, error out=w557:errorcluster)  [unwired: 2 out]
        n160 = Search and Replace String(replace all?=TRUE ("replace all? (F)"), input string=w562, search string=",", replace string="_" ("replace string (\"\")"), error in=w557) -> (result string=w559:string, error out=w556:errorcluster)  [unwired: 3 in, 2 out]
        n161 = Build Array(w559, w579, w578) -> (w574:string[])
        n162 = Insert Into Array(array=w572, index (col)=0 ("index (row)"), new element=w574) -> (w571:string[][])  [unwired: 1 in]
      }
      n163 = Build Array("Instrument Name", "Frequency (GHz)" ("element"), "Power (dBm)" ("element")) -> (w493:string[])
      n164 = Build Path(base path=w450, name or relative path="RFSource_Params.csv") -> (appended path=w478:path)
      n165 = Insert Into Array(array=w497, index (col)=0 ("disabled index (col)"), new element=w493) -> (w474:string[][])  [unwired: 1 in]
      n166 = call-poly <vilib>:"Write Delimited Spreadsheet.vi"("file path (dialog if empty)"=w478, "format (%s)"="%s" ("format (%.3f)"), "2D data"=w474, "error in (no error)"=w473, "transpose? (no:F)"=TRUE, "delimiter (\\t)"="," ("delimiter (\\t)")) -> ("error out"=w453:errorcluster)  [unwired: 8 in, 1 out]
      n167 = Strip Path(path=w450) -> (name=w471:string)  [unwired: 1 out]
      n168 = Unbundle(w472) -> ("DUT"=w470:string, "Ion (ex Kr)"=w469:string, "Board Number"=w468:string, "Effective LET"=w467:string, "Test Type"=w466:T13)  [unwired: 1 out]
      n169 = case shown="\"Single Event Latchup\", Default" w466 {
        tunnel: ["Single Event Latchup (SEL)" "Single Event Transient (SET)"] -> w465
        frame "Single Event Latchup", Default {
        }
        frame "Single Event Transient" {
        }
      }
      n170 = Build Array("Run Number" ("name"), "DUT" ("element"), "Ion" ("element"), "Board Number" ("element"), "Effective LET" ("element"), "Test Type" ("element")) -> (w464:string[])
      n171 = Build Array(w471, w470, w469, w468, w467, w465) -> (w463:string[])
      n172 = Build Array(w464, w463) -> (w451:string[][])
      n173 = Build Path(base path=w450, name or relative path="RunData_Params.csv") -> (appended path=w458:path)
      n174 = call-poly <vilib>:"Write Delimited Spreadsheet.vi"("file path (dialog if empty)"=w458, "format (%s)"="%s" ("format (%.3f)"), "2D data"=w451, "error in (no error)"=w453, "transpose? (no:F)"=TRUE, "delimiter (\\t)"="," ("delimiter (\\t)")) -> ("error out"=w452:errorcluster)  [unwired: 8 in, 1 out]
    }
  }
  "DCPowerInformationClusterArray_Output" <- w41
  "VISAPowerInfoInputOutput" <- w43
  "Run Data SubPanel Output" <- w45
  "Oscilloscope Info Array Output" <- w49
  "Data Was Collected?" <- w38
  "DCPowerInfoArray" <- w37
  "OscilloscopeInfoArray" <- w3
  "RFSourceInfoArray" <- w2
  "RF Subpanel Output" <- w47
  n175 = List Folder(path=w35, pattern="*.txt", error in=w53) -> (path out=w58:path, filenames=w57:string[], error out=w56:errorcluster)  [unwired: 1 in, 1 out]
  n176 = for {
    tunnel: [w648] -> w6
    tunnel: w58 -> [w648]
    tunnel: w57 -> [w650] mode=indexing
    shift-right: [w651] -> w21
    shift-left: w56 -> [w652]
    n177 = Build Path(base path=w648, name or relative path=w650) -> (appended path=w649:path)
    n178 = Delete(path (use dialog)=w649, error in=w652) -> (error out=w651:errorcluster)  [unwired: 3 in, 2 out]
  }
  n179 = Get Date/Time String(date format (0)=enum16{"short", "long", "abbreviated"}."short", seconds (now)=w19, want seconds? (F)=TRUE) -> (date string=w14:string, time string=w15:string)
  n180 = Concatenate Strings(w14, "," ("string"), w15) -> (w13:string)
  n181 = Strip Path(path=w6) -> (name=w62:string)  [unwired: 1 out]
  n182 = Build Path(base path=w6, name or relative path="BeginRecordTimeStamp.txt") -> (appended path=w5:path)
  n183 = Concatenate Strings(w62, "_DCPOWER_COPYFOLDER" ("name or relative path")) -> (w60:string)
  n184 = Open/Create/Replace File(file path (use dialog)=w5, error in=w21, operation (0:open)=T8."open or create", access (0:read/write)=enum16{"read/write", "read-only", "write-only"}."read/write") -> (refnum out=w12:refnum<file>, error out=w20:errorcluster)  [unwired: 2 in, 1 out]
  n185 = Build Path(base path=w6, name or relative path=w60) -> (appended path=w69:path)
  n186 = Write to Text File(file (use dialog)=w12, text=w13, error in=w20) -> (refnum out=w8:refnum<file>, error out=w9:errorcluster)  [unwired: 1 in, 1 out]
  n187 = Close File(refnum=w8, error in=w9) -> (error out=w7:errorcluster)  [unwired: 1 out]
  n188 = Create Folder(path (use dialog)=w69, error in=w7) -> (created path=w64:path, error out=w67:errorcluster)  [unwired: 1 in, 1 out]
  n189 = List Folder(path=w6, error in=w67) -> (path out=w66:path, filenames=w65:string[], error out=w63:errorcluster)  [unwired: 2 in, 1 out]
  n190 = for {
    tunnel: w66 -> [w658]
    tunnel: w65 -> [w657] mode=indexing
    tunnel: w64 -> [w653]
    shift-right: [w660] -> w68
    shift-left: w63 -> [w654]
    tunnel: [w653] -> _
    n191 = Build Path(base path=w658, name or relative path=w657) -> (appended path=w655:path)
    n192 = Build Path(base path=w653, name or relative path=w657) -> (appended path=w656:path)
    n193 = Copy(8:w654, 9:TRUE ("overwrite (F)"), 10:w656, 11:w655) -> (0:w660:errorcluster)  [unwired: 1 in, 2 out]
  }
  "error out" <- w68
